vi "ListaTematy_new.vi"(7 "Jsonconfig":string, 8 "error in (no error)":errorcluster) -> (0 "error out":errorcluster, 2 "data":string[][](array[string]), 3 "Array":string[](array[string]))   [LabVIEW 2017]
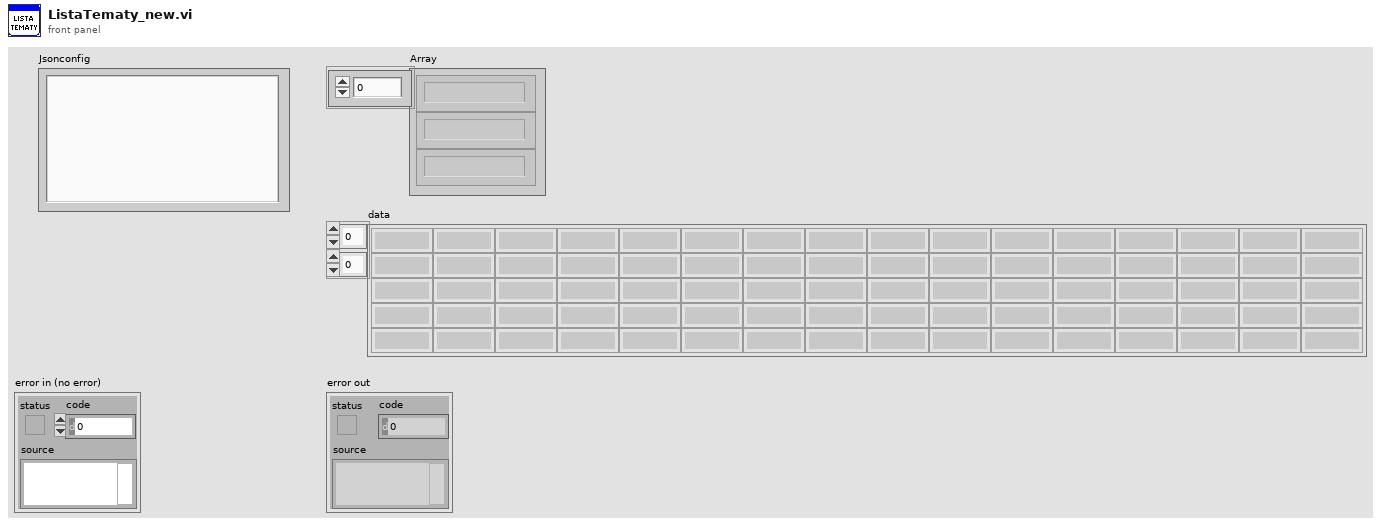
[diagram p1: front panel]
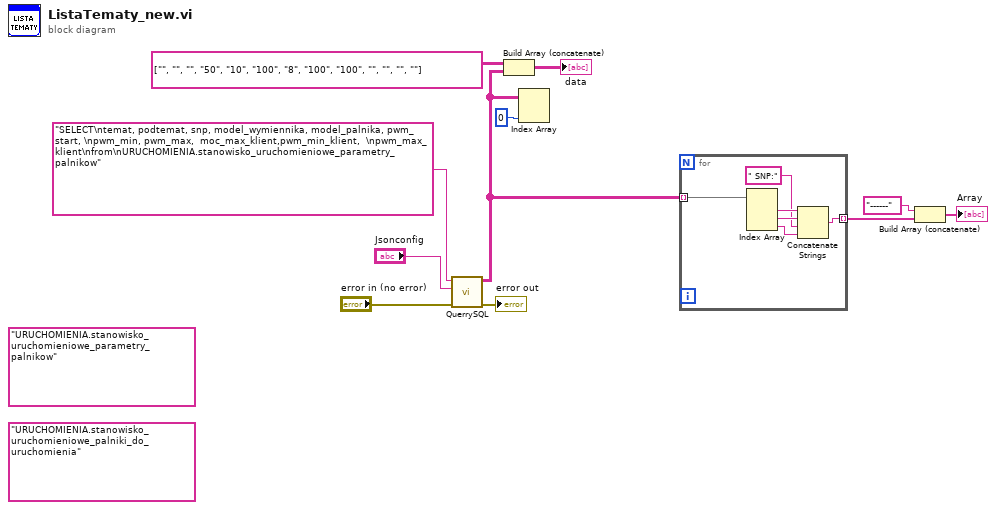
[diagram p0: block diagram]
diagram:
  (unwired) "URUCHOMIENIA.stanowisko_uruchomieniowe_palniki_do_uruchomienia" ("table")
  (unwired) "URUCHOMIENIA.stanowisko_uruchomieniowe_parametry_palnikow" ("table")
  n1 = call "QuerrySQL.vi"("error in (no error)"="error in (no error)", "Jsonconfig"="Jsonconfig", "String"="SELECT\ntemat, podtemat, snp, model_wymiennika, model_palnika, pwm_start, \npwm_min, pwm_max,  moc_max_klient,pwm_min_klient,  \npwm_max_klient\nfrom\nURUCHOMIENIA.stanowisko_uruchomieniowe_parametry_palnikow") -> ("error out"=→"error out":errorcluster, "Array"=w3:string[][])  [unwired: 7 in]
  n2 = Build Array (concatenate)(string[][] [["", "", "", "50", "10", "100", "8", "100", "100", "", "", "", ""]] ("data"), w3) -> (→"data":string[][])
  n3 = Index Array(array=w3, index (col)=0 ("disabled index (col)")) -> ()  [unwired: 1 in, 1 out]
  n4 = for {
    tunnel: w3 -> [w17] mode=indexing
    tunnel: [w15] -> w6 mode=indexing
    n5 = Index Array(array=w17) -> (element #1=w16:string, element #2=w14:string, element #3=w12:string)  [unwired: 3 in]
    n6 = Concatenate Strings(w16, w14, " SNP:" ("string"), w12) -> (w15:string)
  }
  n7 = Build Array (concatenate)("------", w6) -> (→"Array":string[])
